vi "Climb States.vi"() -> ()   [LabVIEW 2018]
panel:
  in  "Climb_Sequence":dbl
  in  "Climber_Sequence_String":string
  in  "Climber_Foot_State":bool
  in  "Climb_Started":bool
  in  "PTO_State":bool
  in  "Climber_Mantis_State":bool
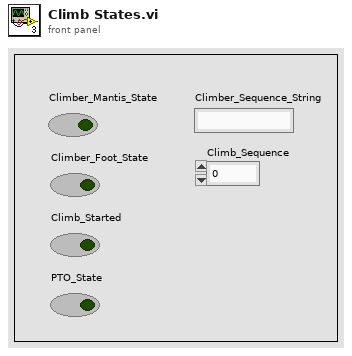
[diagram p1: front panel]
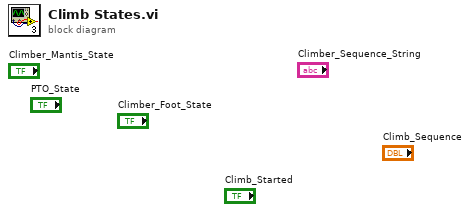
[diagram p0: block diagram]
diagram:
